vi "Replace BD Decoration Text by Label.vi"(8 "error in":errorcluster, 9 "New Content":string, 10 "Label":string, 11 "VI  Ref":refnum<vi>) -> (0 "error out":errorcluster, 1 "Old Content":string, 3 "VI Modified & Saved?":bool)   [LabVIEW 2021, in "Utilities.lvlib"]
doc: "Returns an array of control references and a string array of control label names, from the front panel of the calling VI.\n\nThis VI also accounts for tab controls within other tab controls."
uses:
  Utilities.lvlib
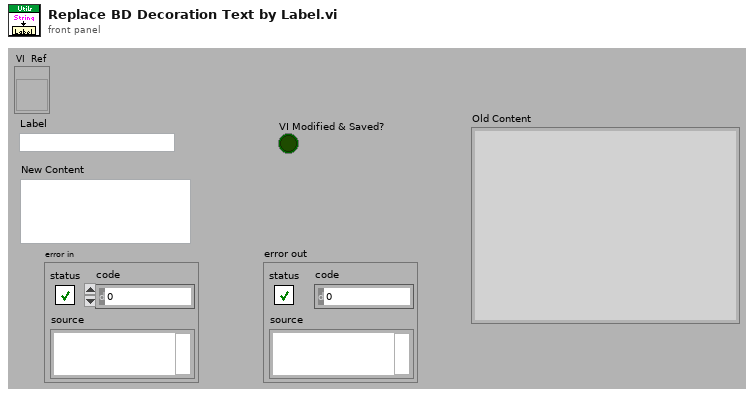
[diagram p1: front panel]
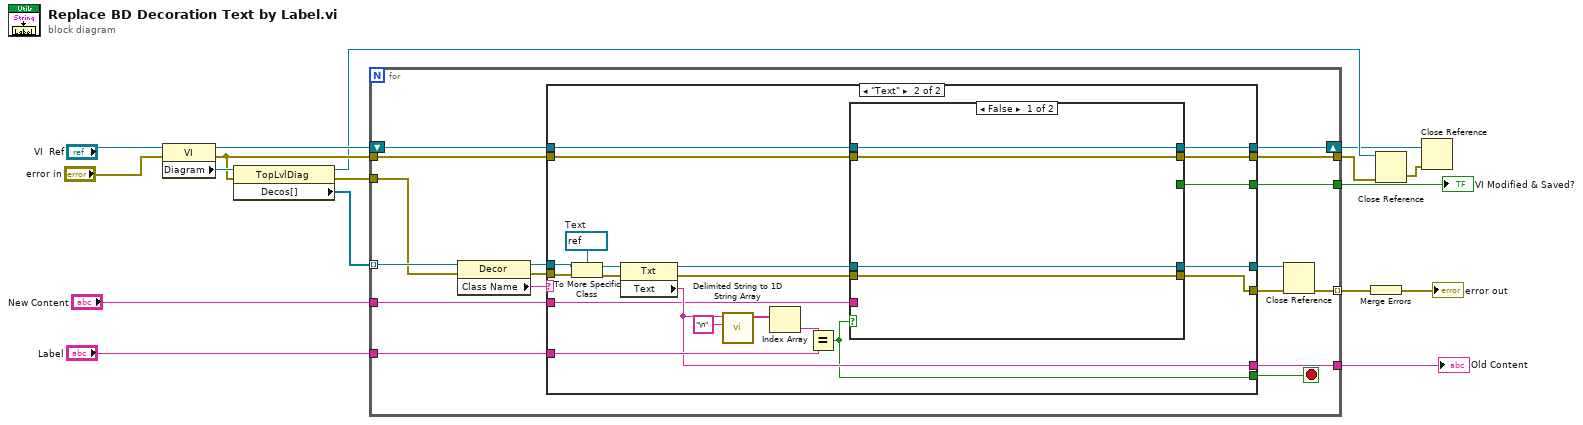
[diagram p0: block diagram]
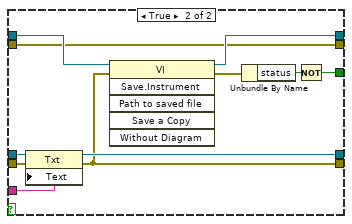
[diagram p3: hidden frame]
diagram:
  n1 = property class="VI"(reference="VI  Ref", error in="error in") -> (reference out=w8:refnum<vi>, error out=w7:errorcluster, "Diagram"=w16:refnum<vi>)
  n2 = property class="TopLvlDiag"(reference=w16, error in=w7) -> (reference out=w4:refnum<vi>, error out=w15:errorcluster, "Decos[]"=w17:refnum<vi>[])
  n3 = for {
    tunnel: "Label" -> [w32]
    tunnel: w17 -> [w28] mode=indexing
    tunnel: w15 -> [w19]
    tunnel: [w29] -> w14 mode=indexing
    tunnel: [w25] -> w10
    tunnel: "New Content" -> [w24]
    tunnel: w7 -> [w22]
    tunnel: [w21] -> w5
    tunnel: [w18] -> w1
    shift-right: [w20] -> w3
    shift-left: w8 -> [w23]
    stop <- w27 stop-if-true
    n4 = property class="Decor"(reference=w28, error in=w19) -> (reference out=w34:refnum<vi>, error out=w33:errorcluster, "Class Name"=w26:string)
    n5 = case shown="\"Text\"" w26 {
      tunnel: w34 -> [w38 w58]
      tunnel: w33 -> [w37 w59]
      tunnel: [w37 w46] -> w30
      tunnel: w32 -> [_ w52]
      tunnel: [w38 w47] -> w31
      tunnel: [_ w45] -> w27
      tunnel: [_ w50] -> w25
      tunnel: w24 -> [_ w44]
      tunnel: w23 -> [w36 w43]
      tunnel: w22 -> [w35 w42]
      tunnel: [_ w41] -> w21
      tunnel: [w36 w40] -> w20
      tunnel: [w35 w39] -> w18
      frame "", Default {
      }
      frame "Text" {
        w57 = refnum<vi> refnum  # Text
        n6 = To More Specific Class(target class=w57, reference=w58, error in=w59) -> (specific class reference=w56:refnum<vi>, error out=w55:errorcluster)
        n7 = property class="Txt"(reference=w56, error in=w55) -> (reference out=w49:refnum<vi>, error out=w48:errorcluster, "Text"=w50:string)
        n8 = call <vilib>:"Delimited String to 1D String Array.vi"("delimiter"="\n", "delimited string"=w50) -> ("string array"=w54:string[])  [unwired: 9 in]
        n9 = Index Array(array=w54) -> (element=w53:string)  [unwired: 1 in]
        n10 = Equal?(x=w53, y=w52) -> (x = y?=w45:bool)
        n11 = case shown="False" w45 {
          tunnel: w49 -> [w63 w74]
          tunnel: w48 -> [w62 w73]
          tunnel: [w63 w69] -> w47
          tunnel: [w62 w68] -> w46
          tunnel: w44 -> [_ w72]
          tunnel: w43 -> [w61 w71]
          tunnel: [w61 w70] -> w40
          tunnel: w42 -> [w60 w64]
          tunnel: [_ w65] -> w41
          tunnel: [w60 w64] -> w39
          frame False {
          }
          frame True {
            n12 = property class="Txt"(reference=w74, error in=w73, "Text"=w72) -> (reference out=w69:refnum<vi>, error out=w68:errorcluster)
            n13 = invoke class="VI" method="Save.Instrument"(reference=w71, error in=w68) -> (reference out=w70:refnum<vi>, error out=w67:errorcluster)  [unwired: 4 in, 4 out]
            n14 = Unbundle By Name(w67) -> ("status"=w66:bool)
            n15 = Not(x=w66) -> (.not. x?=w65:bool)
          }
        }
      }
    }
    n16 = Close Reference(reference=w31, error in (no error)=w30) -> (error out=w29:errorcluster)
  }
  "Old Content" <- w10
  "VI Modified & Saved?" <- w5
  n17 = Merge Errors(w14) -> (→"error out":errorcluster)
  n18 = Close Reference(reference=w4, error in (no error)=w1) -> (error out=w2:errorcluster)
  n19 = Close Reference(reference=w3, error in (no error)=w2) -> ()  [unwired: 1 out]
